vi "save0.vi"(8 "error in (no error)":errorcluster, 9 "base name":string, 10 "folder path":path, 11 "DataCollectionDL110128Streaming in":refnum<class "DataCollectionDL110128Streaming.lvclass">) -> (0 "error out":errorcluster, 3 "DataCollectionDL110128Streaming out":refnum<class "DataCollectionDL110128Streaming.lvclass">)   [LabVIEW 2010, in "DataCollectionDL110128Streaming.lvclass"]
uses:
  DataCollectionDL110128Streaming.lvclass
  DataCollectionDL091104Scaffold/DataCollectionDL091104Scaffold/DataCollectionDL091104Scaffold.lvclass
  DataCollectionDL110128Streaming.lvclass/DataCollectionDL110128Streaming.ctl
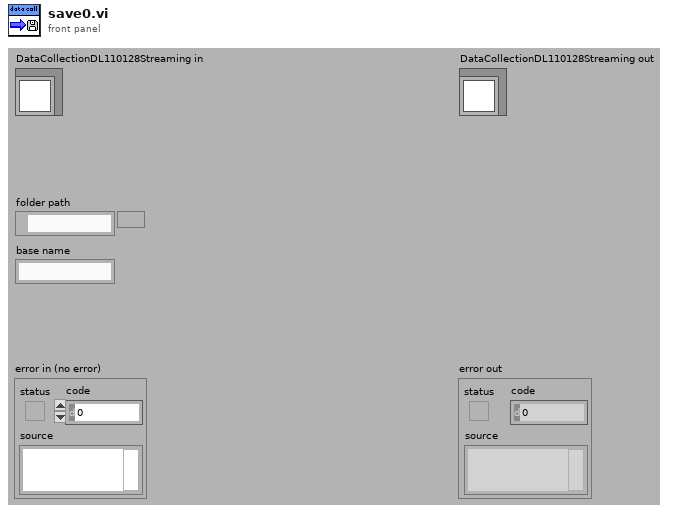
[diagram p1: front panel]
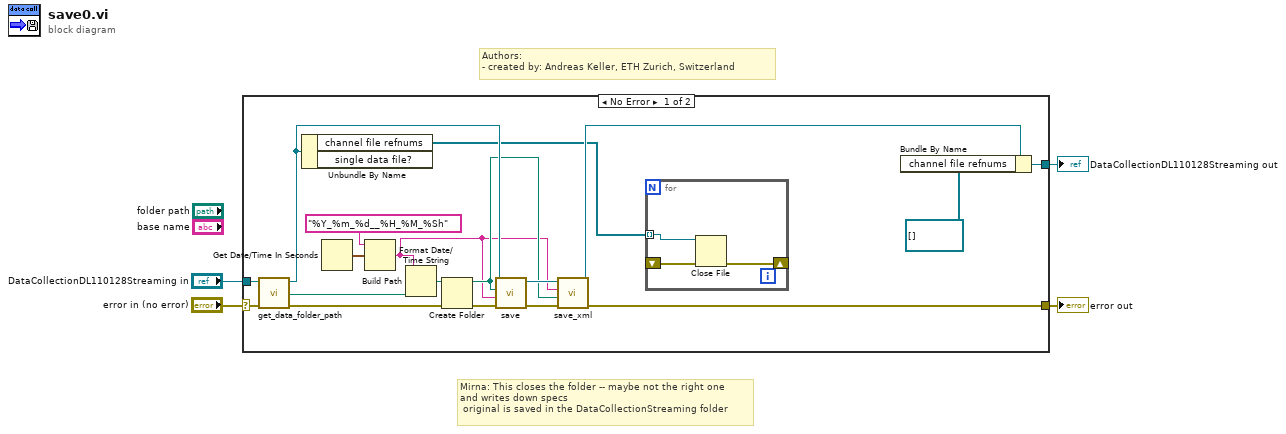
[diagram p0: block diagram]
diagram:
  # "Mirna: This closes the folder -- maybe not the right one\nand writes down specs\n original is saved in the DataCollectionStreaming folder"
  # "Authors: \n- created by: Andreas Keller, ETH Zurich, Switzerland"
  n1 = case shown="No Error" "error in (no error)" {
    selector: "error in (no error)" -> [w22 w27]
    tunnel: [w6 w27] -> w4
    tunnel: [w15 w26] -> w3
    tunnel: "DataCollectionDL110128Streaming in" -> [w21 w26]
    frame No Error {
      n2 = call-dynamic "get_data_folder_path.vi"("error in (no error)"=w22, "GenericComponent in"=w21) -> ("error out"=w16:errorcluster, "data folder path"=w18:path, "GenericComponent out"=w13:refnum<class "DataCollectionDL110128Streaming.lvclass">)  [unwired: 7 out]
      n3 = Unbundle By Name(w13) -> ("channel file refnums"=w5:refnum<file>[])  [unwired: 1 out]
      n4 = Get Date/Time In Seconds() -> (seconds since 1Jan1904=w19:timestamp)
      n5 = Format Date/Time String(time format string (%c)="%Y_%m_%d__%H_%M_%Sh", seconds (now)=w19) -> (date/time string=w8:string)  [unwired: 1 out]
      n6 = Build Path(base path=w18, name or relative path=w8) -> (appended path=w17:path)
      n7 = Create Folder(path (use dialog)=w17, error in=w16) -> (created path=w9:path, error out=w7:errorcluster)  [unwired: 1 in, 1 out]
      n8 = call-parent "save.vi"("error in (no error)"=w7, "base name"=w8, "folder path"=w9, "DL090215DataCollection in"=w13) -> ("error out"=w12:errorcluster, "DL090215DataCollection out"=w11:refnum<class "DataCollectionDL110128Streaming.lvclass">)  [unwired: 6 in]
      n9 = call-dynamic "save_xml.vi"("error in (no error)"=w12, "appended path"=w9, "string"=w8, "DataCollectionDL110128Streaming in"=w11) -> ("error out"=w6:errorcluster, "DataCollectionDL110128Streaming out"=w10:refnum<class "DataCollectionDL110128Streaming.lvclass">)  [unwired: 6 in]
      n10 = for {
        shift-right: [w24] -> _
        shift-left: _ -> [w25]
        tunnel: w5 -> [w23] mode=indexing
        n11 = Close File(refnum=w23, error in=w25) -> (error out=w24:errorcluster)  [unwired: 1 out]
      }
      n12 = Bundle By Name(cluster=w10, "channel file refnums"=refnum<file>[] []) -> (w15:refnum<class "DataCollectionDL110128Streaming.lvclass">)
    }
    frame Error {
    }
  }
  "error out" <- w4
  "DataCollectionDL110128Streaming out" <- w3
